vi "Select Custom Device Dialog.vi"(6 "NIVS.System Definition Root":refnum<k24>, 8 "error in (no error)":errorcluster) -> (0 "error out":errorcluster, 1 "Canceled?":bool, 3 "CD Data":T1)   [LabVIEW 2011]
uses:
  NationalInstruments.VeriStand.SystemStorage
  Dialog Data.ctl
  NationalInstruments.VeriStand.SystemDefinitionAPI
panel:
  in  "Target":u16(ring) items=["Controller"]
  in  "Cancel":bool
  in  "OK":bool
  in  "CD":u16(ring) caption="Custom Device" items=["PXI-2510-3", "PXI-2510-5"]
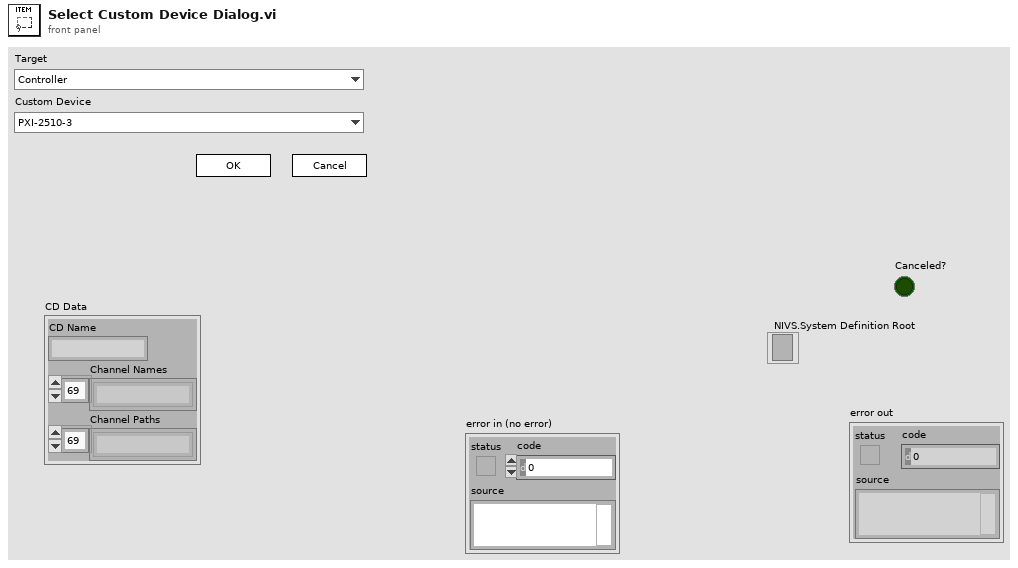
[diagram p1: front panel]
types:
  T1 = cluster{"CD Name":string, "Channel Names":string[], "Channel Paths":string[]}
  T2 = typedef "Dialog Data.ctl" = cluster{"Target Nodes":refnum<k24>[], "Sel Targ Idx":u16, "Sel Targ Node":refnum<k24>, "CD Nodes":refnum<k24>[], "Sel CD Idx":u16, "Sel CD Node":refnum<k24>, "Channel Paths":string[], "Channel Names":string[], "CD Name":string}
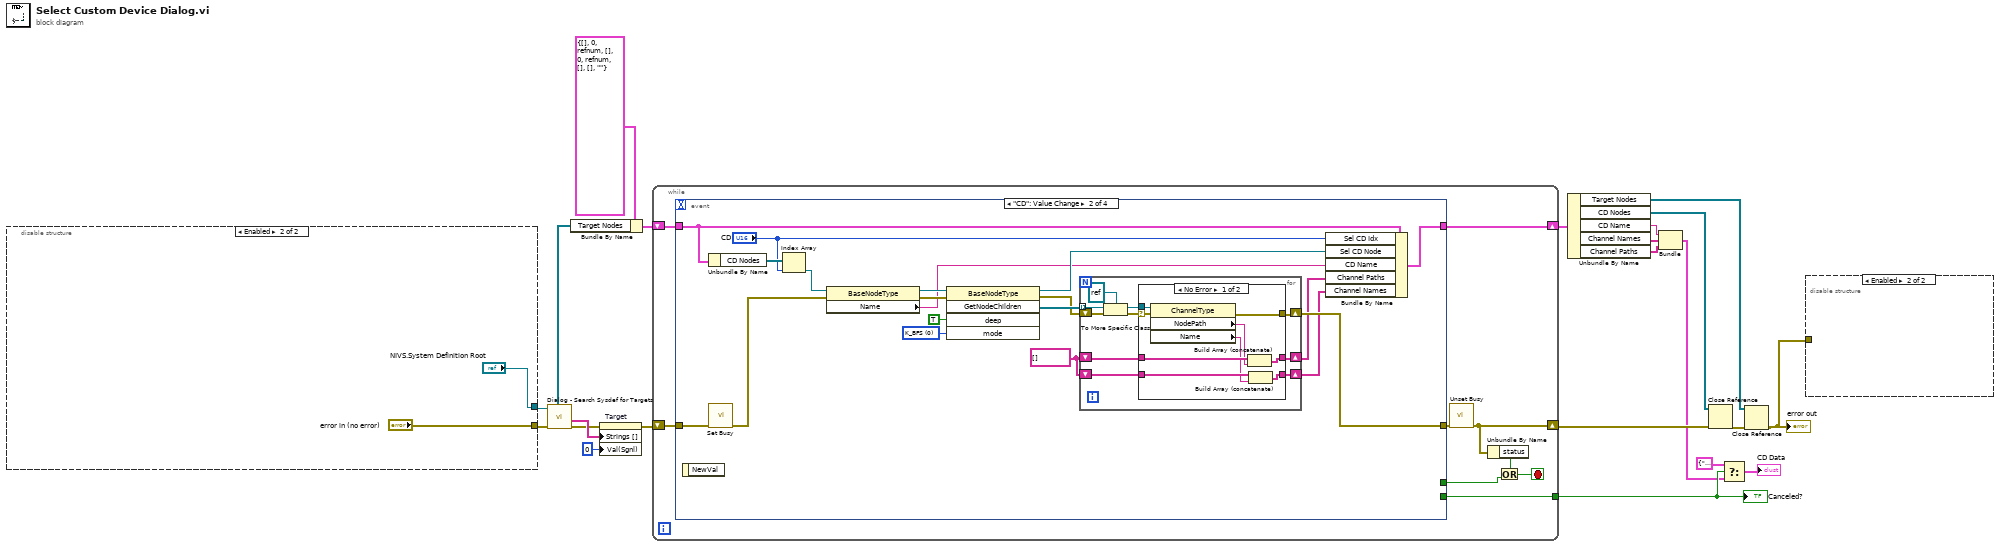
[diagram p0: block diagram]
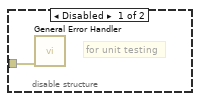
[diagram p2: hidden frame]
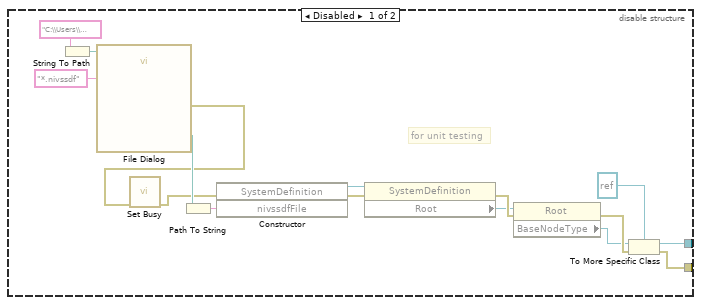
[diagram p3: hidden frame]
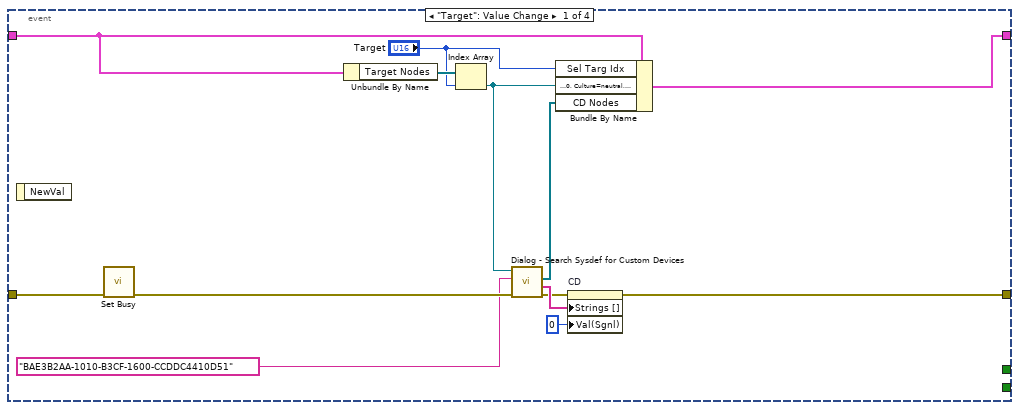
[diagram p4: hidden frame]
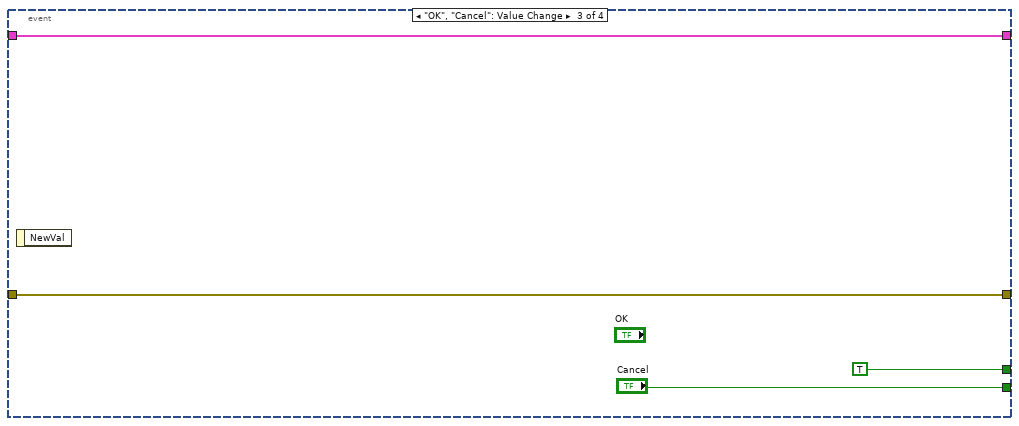
[diagram p6: hidden frame]
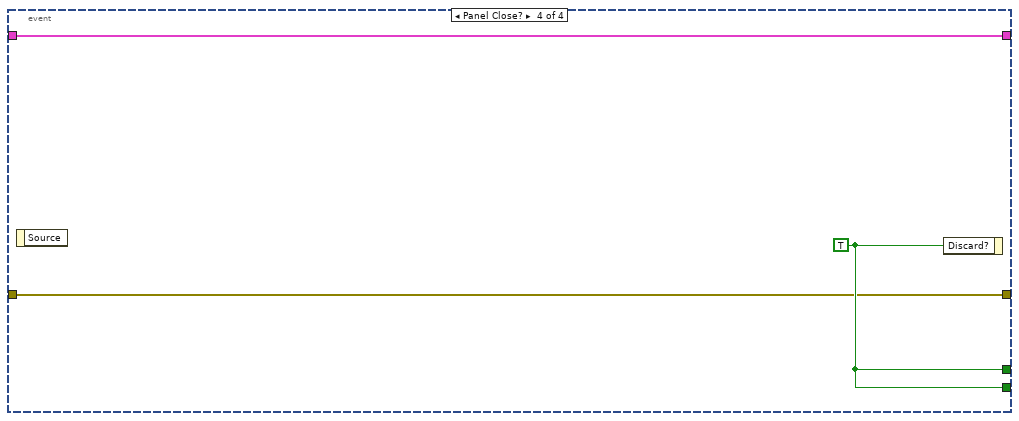
[diagram p7: hidden frame]
diagram:
  n1 = disable-structure shown="Enabled" {
    disable-tunnel: [w24 "NIVS.System Definition Root"] -> w22
    disable-tunnel: [w31 "error in (no error)"] -> w17
    frame Disabled {
      # "for unit testing"
      n2 = String To Path(string="C:\\Users\\Public\\Documents\\National Instruments\\NI VeriStand 2010\\Projects") -> (path=w27:path)
      n3 = call "File Dialog"("start path"=w27, "pattern (all files)"="*.nivssdf") -> ("selected path"=w37:path, "error out"=w25:errorcluster)  [unwired: 10 in, 2 out]
      n4 = call <vilib>:"Set Busy.vi"("error in (no error)"=w25) -> ("error out"=w26:errorcluster)  [unwired: 9 in, 1 out]
      n5 = Path To String(path=w37) -> (string=w36:string)
      n6 = constructor class="SystemDefinition"(error in=w26, "nivssdfFile"=w36) -> (reference out=w34:refnum<k24>, error out=w35:errorcluster)  [unwired: 2 in, 2 out]
      n7 = property class="SystemDefinition"(reference=w34, error in=w35) -> (error out=w33:errorcluster, "Root"=w23:refnum<k24>)  [unwired: 1 out]
      n8 = property class="Root"(reference=w23, error in=w33) -> (error out=w32:errorcluster, "BaseNodeType"=w30:refnum<k24>)  [unwired: 1 out]
      n9 = To More Specific Class(target class=refnum<k24> refnum, reference=w30, error in=w32) -> (specific class reference=w24:refnum<k24>, error out=w31:errorcluster)
    }
    frame Enabled {
    }
  }
  n10 = call "Dialog - Search Sysdef for Targets.vi"("error in (no error)"=w17, "NIVS.System Definition Root"=w22) -> ("error out"=w18:errorcluster, "Target Names"=w21:string[], "Target Nodes"=w11:refnum<k24>[])  [unwired: 6 in, 1 out]
  n11 = Bundle By Name(cluster=T2 {"Target Nodes"=[], "Sel Targ Idx"=0, "Sel Targ Node"=refnum, "CD Nodes"=[], "Sel CD Idx"=0, "Sel CD Node"=refnum, "Channel Paths"=[], "Channel Names"=[], "CD Name"=""} ("Dialog Data"), "Target Nodes"=w11) -> (w12:T2)
  n12 = property on="Target" class="Ring (strict)"(error in=w18, "Strings []"=w21, "Val(Sgnl)"=0 ("index")) -> (error out=w16:errorcluster)  [unwired: 1 in, 1 out]
  n13 = while {
    shift-right: [w43] -> w20
    shift-left: w16 -> [w49]
    tunnel: [w45] -> w7
    shift-right: [w41] -> w10
    shift-left: w12 -> [w42]
    stop <- w48 stop-if-true
    n14 = event shown="[1] \"CD\": Value Change" {
      selector: _ -> [_ _ _ _]
      dyn-events: _ -> [_ _ _ _]
      timeout: _ -> [_ _ _ _]
      tunnel: w49 -> [w61 w81 w106 w108]
      tunnel: [_ _ TRUE w109] -> w46
      tunnel: [w58 w72 w106 w108] -> w44
      tunnel: [_ _ "Cancel" w109] -> w45
      tunnel: w42 -> [w56 w80 w103 w107]
      tunnel: [w55 w79 w103 w107] -> w41
      event "Target": Value Change {
        n15 = event-data() -> ()  [unwired: 1 in, 1 out]
        n16 = call <vilib>:"Set Busy.vi"("error in (no error)"=w61) -> ("error out"=w60:errorcluster)  [unwired: 9 in, 1 out]
        n17 = Unbundle By Name(w56) -> ("Target Nodes"=w54:refnum<k24>[])
        n18 = Index Array(array=w54, index="Target") -> (element=w52:refnum<k24>)
        n19 = call "Dialog - Search Sysdef for Custom Devices.vi"("error in (no error)"=w60, "CD GUID"="BAE3B2AA-1010-B3CF-1600-CCDDC4410D51" ("Demo GUID, pick your own CD's GUID"), "Target Node"=w52) -> ("error out"=w59:errorcluster, "Custom Device Names"=w62:string[], "Custom Device Nodes"=w53:refnum<k24>[])  [unwired: 5 in, 1 out]
        n20 = Bundle By Name(cluster=w56, "Sel Targ Idx"="Target", "Sel Targ Node"=w52, "CD Nodes"=w53) -> (w55:T2)
        n21 = property on="CD" class="Ring (strict)"(error in=w59, "Strings []"=w62, "Val(Sgnl)"=u16 0 ("Value (Signaling)")) -> (error out=w58:errorcluster)  [unwired: 1 in, 1 out]
      }
      event "CD": Value Change {
        w71 = string[] []
        w75 = 0 items=["K_BFS", "K_DFS", "K_CHILDONLY", "K_UP"] ("mode")
        n22 = event-data() -> ()  [unwired: 1 in, 1 out]
        n23 = Unbundle By Name(w80) -> ("CD Nodes"=w78:refnum<k24>[])
        n24 = call <vilib>:"Set Busy.vi"("error in (no error)"=w81) -> ("error out"=w66:errorcluster)  [unwired: 9 in, 1 out]
        n25 = Index Array(array=w78, index="CD") -> (element=w65:refnum<k24>)
        n26 = property class="BaseNodeType"(reference=w65, error in=w66) -> (reference out=w68:refnum<k24>, error out=w67:errorcluster, "Name"=w63:string)
        n27 = invoke class="BaseNodeType" method="GetNodeChildren"(reference=w68, error in=w67, "deep"=TRUE, "mode"=w75) -> (reference out=w64:refnum<k24>, error out=w73:errorcluster, "GetNodeChildren"=w74:refnum<k24>[])  [unwired: 1 in, 2 out]
        n28 = for {
          tunnel: w74 -> [w91] mode=indexing
          shift-right: [w85] -> w72
          shift-left: w73 -> [w90]
          shift-right: [w84] -> w69
          shift-left: w71 -> [w86]
          shift-right: [w82] -> w70
          shift-left: w71 -> [w83]
          n29 = To More Specific Class(target class=refnum<k24> refnum, reference=w91, error in=w90) -> (specific class reference=w87:refnum<k24>, error out=w88:errorcluster)
          n30 = case shown="No Error" w88 {
            selector: w88 -> [w99 _]
            tunnel: w87 -> [w100 _]
            tunnel: w86 -> [w97 w102]
            tunnel: [w98 _] -> w85
            tunnel: [w95 w102] -> w84
            tunnel: w83 -> [w94 w101]
            tunnel: [w92 w101] -> w82
            frame No Error {
              n31 = property class="ChannelType"(reference=w100, error in=w99) -> (error out=w98:errorcluster, "NodePath"=w96:string, "Name"=w93:string)  [unwired: 1 out]
              n32 = Build Array (concatenate)(w97, w96) -> (w95:string[])
              n33 = Build Array (concatenate)(w94, w93) -> (w92:string[])
            }
            frame Error {
            }
          }
        }
        n34 = Bundle By Name(cluster=w80, "Sel CD Idx"="CD", "Sel CD Node"=w64, "CD Name"=w63, "Channel Paths"=w69, "Channel Names"=w70) -> (w79:T2)
      }
      event "OK", "Cancel": Value Change {
        n35 = event-data() -> ()  [unwired: 1 in, 1 out]
      }
      event Panel Close? {
        w109 = TRUE ("Discard?")
        n36 = event-data() -> ()  [unwired: 1 in, 1 out]
        n37 = event-data("Discard?"=w109) -> ()  [unwired: 1 in, 1 out]
      }
    }
    n38 = call <vilib>:"Unset Busy.vi"("error in (no error)"=w44) -> ("error out"=w43:errorcluster)  [unwired: 10 in]
    n39 = Unbundle By Name(w43) -> ("status"=w47:bool)
    n40 = Or(x=w47, y=w46) -> (x .or. y?=w48:bool)
  }
  "Canceled?" <- w7
  n41 = Unbundle By Name(w10) -> ("Target Nodes"=w8:refnum<k24>[], "CD Nodes"=w9:refnum<k24>[], "CD Name"=w6:string, "Channel Names"=w5:string[], "Channel Paths"=w4:string[])
  n42 = Bundle("CD Name"=w6, "Channel Names"=w5, "Channel Paths"=w4) -> (w2:T1)  [unwired: 1 in]
  n43 = Close Reference(reference=w9, error in (no error)=w20) -> (error out=w19:errorcluster)
  n44 = Select(t=T1 {"CD Name"="", "Channel Names"=[], "Channel Paths"=[]} ("output cluster"), s=w7, f=w2) -> (s? t:f=→"CD Data":T1)
  n45 = Close Reference(reference=w8, error in (no error)=w19) -> (error out=w15:errorcluster)
  "error out" <- w15
  n46 = disable-structure shown="Enabled" {
    disable-tunnel: w15 -> [w110 _]
    frame Disabled {
      # "for unit testing"
      n47 = call <vilib>:"General Error Handler.vi"("error in (no error)"=w110) -> ()  [unwired: 10 in, 5 out]
    }
    frame Enabled {
    }
  }
